vi "Init Virtual Instruments.vi"(8 "error in":errorcluster, 10 "Virt Instrs":T1(array[cluster]), 11 "MSS Target Actor in":refnum<class "MSS Target Actor.lvclass">) -> (0 "error out":errorcluster, 3 "MSS Target Actor out":refnum<class "MSS Target Actor.lvclass">)   [LabVIEW 2023, in "MSS Target Actor.lvlib" / "MSS Target Actor.lvclass"]
uses:
  MSS Target Actor.lvclass
  MSS Target Actor.lvclass/MSS Target Actor.ctl
  Measure and Stimulus Subsystems/Measure and Stimulus Subsystems.lvclass
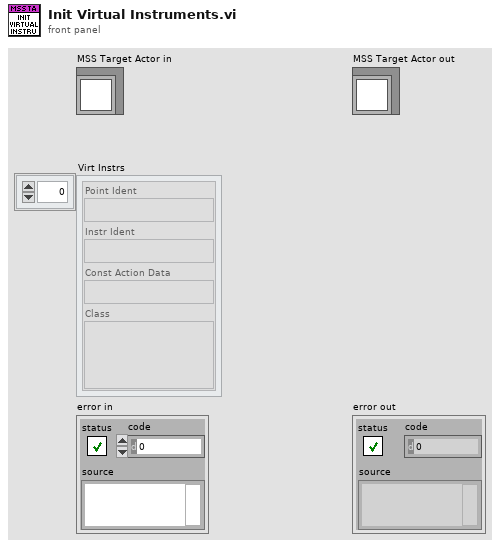
[diagram p1: front panel]
types:
  T1 = cluster{"Point Ident":string, "Instr Ident":string, "Const Action Data":string, "Class":string}[]
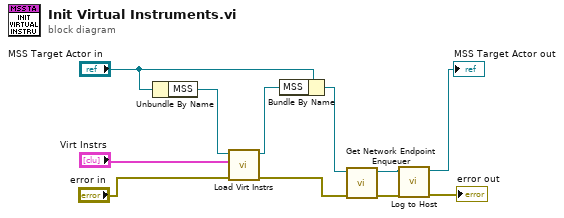
[diagram p0: block diagram]
diagram:
  n1 = Unbundle By Name("MSS Target Actor in") -> ("MSS"=w11:refnum<class "Measure and Stimulus Subsystems.lvclass">)
  n2 = call "Load Virt Instrs.vi"("error in"="error in", "Virt Instrs"="Virt Instrs", "MSS in"=w11) -> ("error out"=w4:errorcluster, "MSS out"=w10:refnum<class "Measure and Stimulus Subsystems.lvclass">)  [unwired: 7 in]
  n3 = Bundle By Name(cluster="MSS Target Actor in", "MSS"=w10) -> (w3:refnum<class "MSS Target Actor.lvclass">)
  n4 = call "Get Network Endpoint Enqueuer.vi"("error in"=w4, "MSS Target Actor in"=w3) -> ("error out"=w6:errorcluster, "MSS Target Actor out"=w2:refnum<class "MSS Target Actor.lvclass">)  [unwired: 6 in, 2 out]
  n5 = call "Log to Host.vi"("error in"=w6, "MSS Target Actor in"=w2) -> ("error out"=→"error out":errorcluster, "MSS Target Actor out"=→"MSS Target Actor out":refnum<class "MSS Target Actor.lvclass">)  [unwired: 8 in]
